vi "Signed to Unsigned.vi"(1 "Symbol In":i32[](array[numeric]), 2 "QAM Complexity":T1(ring)) -> (0 "BitStream Out":i32[](array[numeric]))   [LabVIEW 2018]
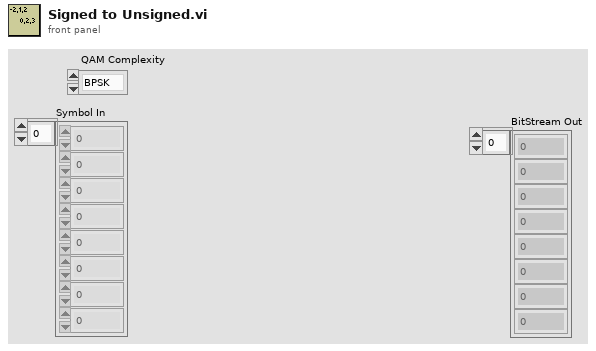
[diagram p1: front panel]
types:
  T1 = enum16{"BPSK", "QPSK", "16-QAM", "64-QAM", "256-QAM"}
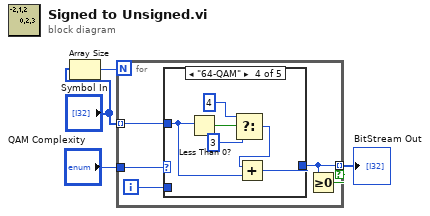
[diagram p0: block diagram]
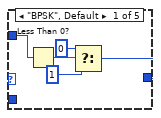
[diagram p2: hidden frame]
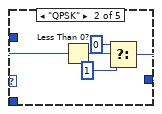
[diagram p3: hidden frame]
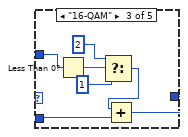
[diagram p4: hidden frame]
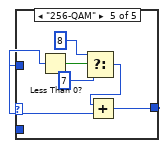
[diagram p5: hidden frame]
diagram:
  n1 = Array Size(array="Symbol In") -> (size(s)=w4:i32)
  n2 = for {
    N: w4 -> [_]
    tunnel: "QAM Complexity" -> [w9]
    tunnel: "Symbol In" -> [w7] mode=indexing
    tunnel: [w5] -> w1 mode=indexing if=w6
    i -> [w8]
    n3 = case shown="\"64-QAM\"" w9 {
      tunnel: w8 -> [_ _ _ _ _]
      tunnel: w7 -> [w14 w15 w20 w26 w32]
      tunnel: [w12 w16 w22 w27 w33] -> w5
      frame "BPSK", Default {
        n4 = Less Than 0?(x=w14) -> (x < 0?=w13:bool)
        n5 = Select(t=0, s=w13, f=1) -> (s? t:f=w12:i32)
      }
      frame "QPSK" {
        n6 = Less Than 0?(x=w15) -> (x < 0?=w19:bool)
        n7 = Select(t=0, s=w19, f=1) -> (s? t:f=w16:i32)
      }
      frame "16-QAM" {
        n8 = Less Than 0?(x=w20) -> (x < 0?=w25:bool)
        n9 = Select(t=2, s=w25, f=1) -> (s? t:f=w21:i32)
        n10 = Add(x=w21, y=w20) -> (x+y=w22:i32)
      }
      frame "64-QAM" {
        n11 = Less Than 0?(x=w26) -> (x < 0?=w31:bool)
        n12 = Select(t=4, s=w31, f=3) -> (s? t:f=w28:i32)
        n13 = Add(x=w28, y=w26) -> (x+y=w27:i32)
      }
      frame "256-QAM" {
        n14 = Less Than 0?(x=w32) -> (x < 0?=w37:bool)
        n15 = Select(t=8, s=w37, f=7) -> (s? t:f=w34:i32)
        n16 = Add(x=w34, y=w32) -> (x+y=w33:i32)
      }
    }
    n17 = Greater Or Equal To 0?(x=w5) -> (x >= 0?=w6:bool)
  }
  "BitStream Out" <- w1
